vi "Max Errors.vi"(1 "stop":bool, 2 "error":bool) -> (0 "Cont?":bool)   [LabVIEW 2024]
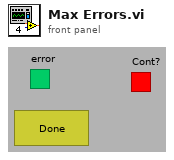
[diagram p1: front panel]
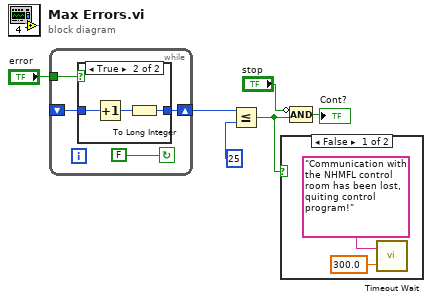
[diagram p0: block diagram]
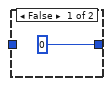
[diagram p2: hidden frame]
diagram:
  n1 = while {
    tunnel: "error" -> [w10]
    shift-left: _ -> [w8]
    shift-right: [w9] -> w5
    stop <- FALSE continue-if-true
    n2 = case shown="True" w10 {
      tunnel: [0 w12] -> w9
      tunnel: w8 -> [_ w14]
      frame False {
      }
      frame True {
        n3 = Increment(x=w14) -> (x+1=w13:i32)
        n4 = To Long Integer(number=w13) -> (32bit integer=w12:i32)
      }
    }
  }
  n5 = Less Or Equal?(x=w5, y=25) -> (x <= y?=w3:bool)
  n6 = case shown="False" w3 {
    frame False {
      n7 = call "Timeout Wait.vi"("Seconds to timeout"=300.0, "Message"="Communication with the NHMFL control room has been lost, quiting control program!" ("message")) -> ()
    }
    frame True {
    }
  }
  n8 = Compound Arithmetic op=AND(invert "stop", w3) -> (→"Cont?":bool)
